vi "Build Preview String.vi"(8 "error in (no error)":errorcluster, 10 "last checked time stamp":timestamp, 11 "Feed in":refnum<class "Feed.lvclass">) -> (0 "error out":errorcluster, 1 "new item count":i32, 2 "preview string":string, 3 "Feed out":refnum<class "Feed.lvclass">)   [LabVIEW 2017, in "Feed.lvclass"]
uses:
  <vilib>/NI_RSS/Feed/Feed.lvclass
  <vilib>/NI_RSS/FeedItem/FeedItem.lvclass
panel:
  in  "More string":string="\nMore..."
  in  "bullet":string=" - "
  in  "String":string="Latest articles:\n"
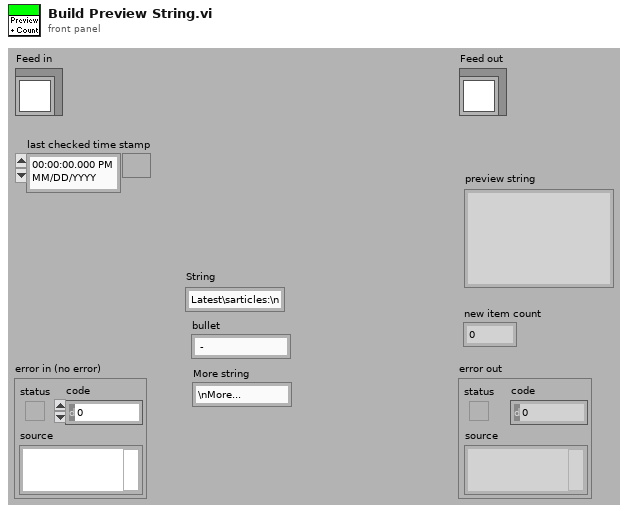
[diagram p1: front panel]
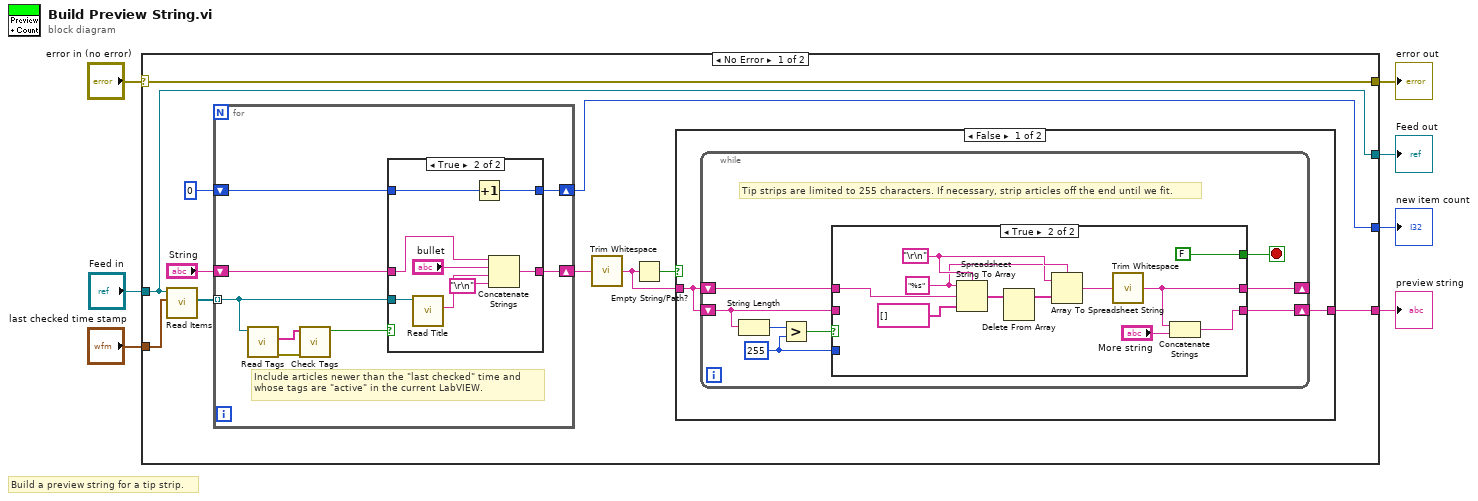
[diagram p0: block diagram]
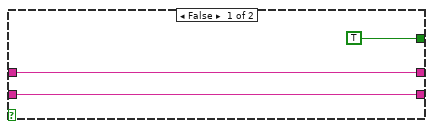
[diagram p2: hidden frame]
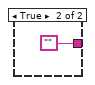
[diagram p3: hidden frame]
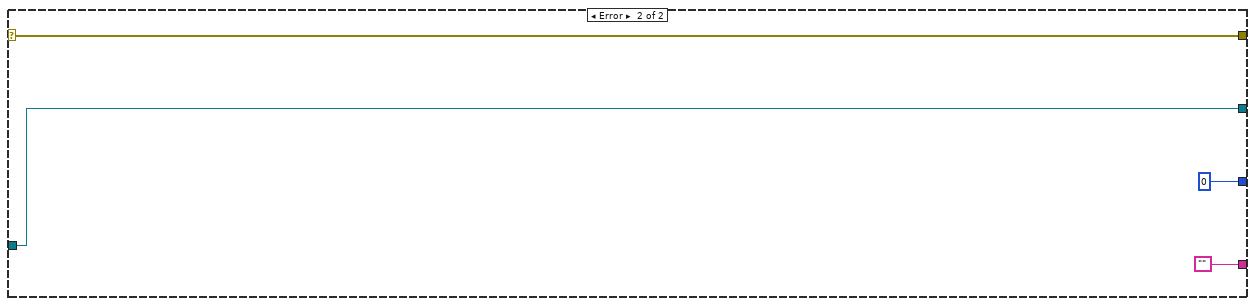
[diagram p5: hidden frame]
diagram:
  # "Build a preview string for a tip strip."
  n1 = case shown="No Error" "error in (no error)" {
    selector: "error in (no error)" -> [w18 w65]
    tunnel: [w18 w65] -> w6
    tunnel: [w17 w64] -> w4
    tunnel: "Feed in" -> [w17 w64]
    tunnel: "last checked time stamp" -> [w8 _]
    tunnel: [w12 0] -> w2
    tunnel: [w11 ""] -> w1
    frame No Error {
      n2 = call-dynamic "Read Items.vi"("After (all)"=w8, "Feed.lvclass in"=w17) -> ("Items"=w16:refnum<class "FeedItem.lvclass">[])  [unwired: 1 in, 8 out]
      n3 = for {
        tunnel: w16 -> [w47] mode=indexing
        shift-right: [w50] -> w12
        shift-left: 0 -> [w51]
        shift-right: [w48] -> w13
        shift-left: "String" -> [w49]
        # "Include articles newer than the \"last checked\" time and\nwhose tags are \"active\" in the current LabVIEW."
        n4 = call-dynamic "Read Tags.vi"("FeedItem.lvclass in"=w47) -> ("error out"=w45:errorcluster, "Tags"=w46:string[])  [unwired: 1 in, 8 out]
        n5 = call <vilib>:"Check Tags.vi"("error in (no error)"=w45, "Tags"=w46) -> ("active"=w44:bool)  [unwired: 9 out]
        n6 = case shown="True" w44 {
          tunnel: w51 -> [w53 w59]
          tunnel: [w53 w61] -> w50
          tunnel: w49 -> [w52 w58]
          tunnel: [w52 w60] -> w48
          tunnel: w47 -> [_ w57]
          frame False {
          }
          frame True {
            n7 = call-dynamic "Read Title.vi"("FeedItem.lvclass in"=w57) -> ("Title"=w54:string)  [unwired: 1 in, 9 out]
            n8 = Increment(x=w59) -> (x+1=w61:i32)
            n9 = Concatenate Strings(w58, "bullet", w54, "\r\n") -> (w60:string)
          }
        }
      }
      n10 = call <vilib>:"Trim Whitespace.vi"("string"=w13) -> ("trimmed string"=w10:string)  [unwired: 1 in]
      n11 = Empty String/Path?(string/path=w10) -> (empty?=w9:bool)
      n12 = case shown="False" w9 {
        tunnel: [w20 ""] -> w11
        tunnel: w10 -> [w19 _]
        frame False {
          n13 = while {
            shift-right: [w25] -> w20
            shift-left: w19 -> [w23]
            shift-right: [w22] -> _
            shift-left: w19 -> [w24]
            stop <- w21 stop-if-true
            w27 = 255 ("y")
            # "Tip strips are limited to 255 characters. If necessary, strip articles off the end until we fit."
            n14 = String Length(string=w23) -> (length=w28:i32)
            n15 = Greater?(x=w28, y=w27) -> (0:w26:bool)
            n16 = case shown="True" w26 {
              tunnel: w27 -> [_ _]
              tunnel: [w31 w41] -> w25
              tunnel: w24 -> [w30 w38]
              tunnel: w23 -> [w31 _]
              tunnel: [w30 w32] -> w22
              tunnel: [TRUE FALSE] -> w21
              frame False {
              }
              frame True {
                w34 = "%s" ("format string")
                w36 = "\r\n"
                n17 = Spreadsheet String To Array(delimiter (Tab)=w36, format string=w34, spreadsheet string=w38, array type (2D Dbl)=string[] []) -> (array=w39:string[])
                n18 = Delete From Array(array=w39) -> (array with subset deleted=w37:string[])  [unwired: 2 in, 1 out]
                n19 = Array To Spreadsheet String(delimiter (Tab)=w36, array=w37, 3:w34) -> (spreadsheet string=w35:string)
                n20 = call <vilib>:"Trim Whitespace.vi"("string"=w35) -> ("trimmed string"=w32:string)  [unwired: 1 in]
                n21 = Concatenate Strings(w32, "More string") -> (w41:string)
              }
            }
          }
        }
        frame True {
        }
      }
    }
    frame Error {
    }
  }
  "error out" <- w6
  "Feed out" <- w4
  "preview string" <- w1
  "new item count" <- w2
